vi "SwerveDrivePoseEst_AddVisionMeasurement.vi"(9 "TImeStamp_Seconds":dbl=0.02, 10 "visionRobotPose":T10={"TRANSLATION"={"X"=0.0, "Y"=0.0}, "ROTATION"={"VALUE"=0.0, "COS"=1.0, "SIN"=0.0}} {"ROTATION"."SIN" format="%13.4f"; "ROTATION"."COS" format="%13.4f"; "ROTATION"."VALUE" format="%13.4f"; "TRANSLATION"."Y" format="%14.3f"; "TRANSLATION"."X" format="%14.3f"}, 11 "in SwerveDrivePoseEstimate":T2={"M_VisionContR"=[], "m_nominal_dT"=0.0, "m_PrevTime_Sec"=0.0, "m_GyroOffset"={"VALUE"=0.0, "COS"=1.0, "SIN"=0.0}, "m_PrevAngle"={"VALUE"=0.0, "COS"=1.0, "SIN"=0.0}, "m_Observer"={"m_P"=[], "m_xHat"=[], "States"=0, "Outputs"=0, "m_ContR"=[], "m_ContQ"=[], "m_SigmasF"=[], "m_dT_Sec"=0.0, "MERWE_SCALED_SIGMA_PTS"={"m_Wm"=[], "States"=0, "Alpha"=0.0, "m_Wc"=[], "Kappa"=0}, "meanFuncX"=refnum, "meanFuncY"=refnum, "residualFuncX"=refnum, "residualFuncY"=refnum, "addFuncX"=refnum, "addFuncXExtra"=variant, "residualFuncYExtra"=variant, "residualFuncXExtra"=variant, "MeanFuncYExtra"=variant, "MeanFuncXExtra"=variant, "Inputs"=0}, "m_kinematics"={"NumModules"=0, "InverseKinematics"=[], "ForwardKinematics"=[], "Modules"=[], "PrevCoR"={"X"=0.0, "Y"=0.0}}, "Pose_Buffer"={"TimeStamps"=[], "Pose"=[], "Min_TimeStamp"=0.0, "Max_TimeStamp"=0.0, "ItemCount"=0, "MaxBufferTime"=0.0}} {"Pose_Buffer"."Pose"."ROTATION"."SIN" format="%13.4f"; "Pose_Buffer"."Pose"."ROTATION"."COS" format="%13.4f"; "Pose_Buffer"."Pose"."ROTATION"."VALUE" format="%13.4f"; "Pose_Buffer"."Pose"."TRANSLATION"."Y" format="%14.3f"; "Pose_Buffer"."Pose"."TRANSLATION"."X" format="%14.3f"; "m_kinematics"."PrevCoR"."Y" format="%14.3f"; "m_kinematics"."PrevCoR"."X" format="%14.3f"; "m_kinematics"."Modules"."Y" format="%14.3f"; "m_kinematics"."Modules"."X" format="%14.3f"; "m_PrevAngle"."SIN" format="%13.4f"; "m_PrevAngle"."COS" format="%13.4f"; "m_PrevAngle"."VALUE" format="%13.4f"; "m_GyroOffset"."SIN" format="%13.4f"; "m_GyroOffset"."COS" format="%13.4f"; "m_GyroOffset"."VALUE" format="%13.4f"}) -> (0 "Error":bool, 3 "OutSwerveDrivePoseEstimate":T2={"M_VisionContR"=[], "m_nominal_dT"=0.0, "m_PrevTime_Sec"=0.0, "m_GyroOffset"={"VALUE"=0.0, "COS"=1.0, "SIN"=0.0}, "m_PrevAngle"={"VALUE"=0.0, "COS"=1.0, "SIN"=0.0}, "m_Observer"={"m_P"=[], "m_xHat"=[], "States"=0, "Outputs"=0, "m_ContR"=[], "m_ContQ"=[], "m_SigmasF"=[], "m_dT_Sec"=0.0, "MERWE_SCALED_SIGMA_PTS"={"m_Wm"=[], "States"=0, "Alpha"=0.0, "m_Wc"=[], "Kappa"=0}, "meanFuncX"=refnum, "meanFuncY"=refnum, "residualFuncX"=refnum, "residualFuncY"=refnum, "addFuncX"=refnum, "addFuncXExtra"=variant, "residualFuncYExtra"=variant, "residualFuncXExtra"=variant, "MeanFuncYExtra"=variant, "MeanFuncXExtra"=variant, "Inputs"=0}, "m_kinematics"={"NumModules"=0, "InverseKinematics"=[], "ForwardKinematics"=[], "Modules"=[], "PrevCoR"={"X"=0.0, "Y"=0.0}}, "Pose_Buffer"={"TimeStamps"=[], "Pose"=[], "Min_TimeStamp"=0.0, "Max_TimeStamp"=0.0, "ItemCount"=0, "MaxBufferTime"=0.0}} {"Pose_Buffer"."Pose"."ROTATION"."SIN" format="%13.4f"; "Pose_Buffer"."Pose"."ROTATION"."COS" format="%13.4f"; "Pose_Buffer"."Pose"."ROTATION"."VALUE" format="%13.4f"; "Pose_Buffer"."Pose"."TRANSLATION"."Y" format="%14.3f"; "Pose_Buffer"."Pose"."TRANSLATION"."X" format="%14.3f"; "m_kinematics"."PrevCoR"."Y" format="%14.3f"; "m_kinematics"."PrevCoR"."X" format="%14.3f"; "m_kinematics"."Modules"."Y" format="%14.3f"; "m_kinematics"."Modules"."X" format="%14.3f"; "m_PrevAngle"."SIN" format="%13.4f"; "m_PrevAngle"."COS" format="%13.4f"; "m_PrevAngle"."VALUE" format="%13.4f"; "m_GyroOffset"."SIN" format="%13.4f"; "m_GyroOffset"."COS" format="%13.4f"; "m_GyroOffset"."VALUE" format="%13.4f"})   [LabVIEW 2019, in "Trajectory_Library.lvlib"]
doc: "Add a vision measurement to the Unscented Kalman Filter. This will correct the odometry pose estimate while still accounting for measurement noise.\n \nThis method can be called as infrequently as you want, as long as you are calling SwerveDrivePoseEstimator_update every loop.\n\nTo promote stability of the pose estimate and make it robust to bad vision data, we recommend only adding vision measurements that are already within one meter or so of the current pose estimate.\n \nInputs:\n - SwervePoseEst -- Data cluster containing SwervePoseEst data\n - visionRobotPoseMeters -- The pose of the robot as measured \n by the vision camera.\n - timestampSeconds -- The timestamp of the vision measurement in \n seconds. Note that if you don't use your own time \n source by calling SwerveDrivePoseEstimator_updateWithTime\n then you must use a timestamp with an epoch since FPGA \n startup (i.e. the epoch of this timestamp is the same \n epoch as Timer.getFPGATimestamp.) This means that you \n should use Timer.getFPGATimestamp as your time source or \n sync the epochs.\n\nOutputs:\n - outSwevePoseEst -- Updated data cluster \n - Error -- If TRUE, an error occured."
uses:
  Trajectory_Library.lvlib
  SWERVE_DRIVE_POSE_EST.ctl
  <vilib>/Analysis/Matrix/Datatypes/RealMatrix.ctl
  ROTATION2D.ctl
  UNSCENTED_KALMAN_FILTER.ctl
  MERWE_SCALED_SIGMA_PTS.ctl
  CALLBACK_FUNC_TYPE.ctl
  SWERVE_DRIVE_KINEMATICS.ctl
  TRANSLATION2D.ctl
  TIME_INTERPOLATABLE_POSE.ctl
  POSE2D.ctl
  Pose2d_RelativeTo.vi
  Transform2d_Create_TransRot.vi
  Translation2d_RotateBy.vi
  Translation2d_Plus.vi
  Rotation2d_Plus.vi
  Pose2d_New_TRRO.vi
  VecBuilder_3x1Fill.vi
  Pose2d_getXYAngle.vi
  Transform2d_Create_PosePose.vi
  Translation2d_Create.vi
  Rotation2d_RotateBy.vi
  Rotation2d_UnaryMinus.vi
  Translation2d_Minus.vi
  Rotation2d_Minus.vi
  Rotation2d_CreateXY.vi
  Rotation2d_CreateAngle.vi
  Util_CalcDist.vi
  <vilib>/Analysis/Matrix/NI_Matrix.lvlib
panel:
  in  "Cluster":cluster{"VisionDiscreteR":T1}
  # "<3, 3>"
  # "State Estimate <Statess,1>"
  # "<States, States>"
  # "<States, ?>"
  # "<Statess,  States>"
  # "<Outputs, Outputs>"
  # "<?, 1>"
  # "<?, 1>"
  # "<3, 3>"
  # "State Estimate <Statess,1>"
  # "<States, States>"
  # "<States, ?>"
  # "<Statess,  States>"
  # "<Outputs, Outputs>"
  # "<?, 1>"
  # "<?, 1>"
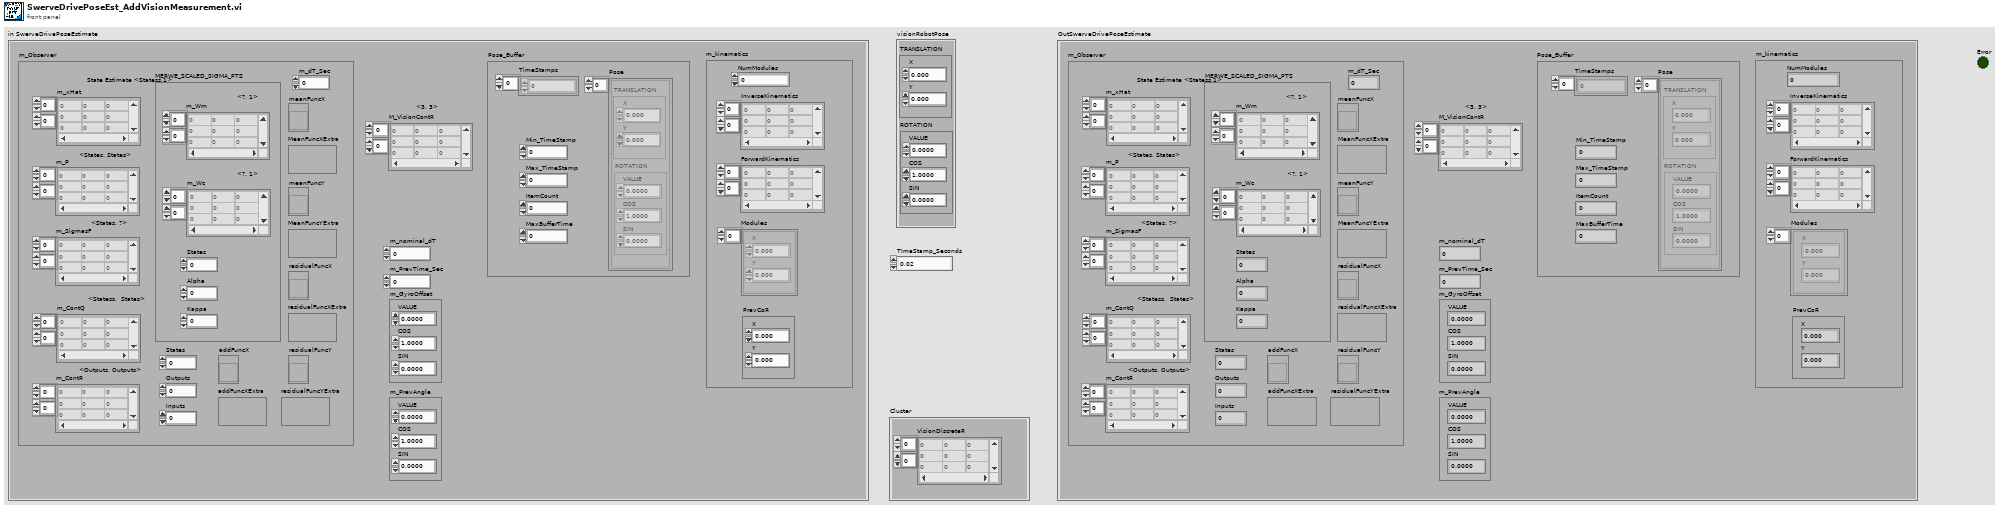
[diagram p1: front panel]
types:
  T1 = typedef "NI_Matrix.lvlib/RealMatrix.ctl" = dbl[][]
  T2 = typedef "Trajectory_Library.lvlib/SWERVE_DRIVE_POSE_EST.ctl" = cluster{"M_VisionContR":T1, "m_nominal_dT":dbl, "m_PrevTime_Sec":dbl, "m_GyroOffset":T3, "m_PrevAngle":T3, "m_Observer":T4, "m_kinematics":T7, "Pose_Buffer":T9}
  T3 = typedef "Trajectory_Library.lvlib/ROTATION2D.ctl" = cluster{"VALUE":dbl, "COS":dbl, "SIN":dbl}
  T4 = typedef "Trajectory_Library.lvlib/UNSCENTED_KALMAN_FILTER.ctl" = cluster{"m_P":T1, "m_xHat":T1, "States":i32, "Outputs":i32, "m_ContR":T1, "m_ContQ":T1, "m_SigmasF":T1, "m_dT_Sec":dbl, "MERWE_SCALED_SIGMA_PTS":T5, "meanFuncX":T6, "meanFuncY":T6, "residualFuncX":T6, "residualFuncY":T6, "addFuncX":T6, "addFuncXExtra":variant, "residualFuncYExtra":variant, "residualFuncXExtra":variant, "MeanFuncYExtra":variant, "MeanFuncXExtra":variant, "Inputs":i32}
  T5 = typedef "Trajectory_Library.lvlib/MERWE_SCALED_SIGMA_PTS.ctl" = cluster{"m_Wm":T1, "States":i32, "Alpha":dbl, "m_Wc":T1, "Kappa":i32}
  T6 = typedef "Trajectory_Library.lvlib/CALLBACK_FUNC_TYPE.ctl" = refnum<vi>
  T7 = typedef "Trajectory_Library.lvlib/SWERVE_DRIVE_KINEMATICS.ctl" = cluster{"NumModules":i32, "InverseKinematics":T1, "ForwardKinematics":T1, "Modules":T8[], "PrevCoR":T8}
  T8 = typedef "Trajectory_Library.lvlib/TRANSLATION2D.ctl" = cluster{"X":dbl, "Y":dbl}
  T9 = typedef "Trajectory_Library.lvlib/TIME_INTERPOLATABLE_POSE.ctl" = cluster{"TimeStamps":dbl[], "Pose":T10[], "Min_TimeStamp":dbl, "Max_TimeStamp":dbl, "ItemCount":i32, "MaxBufferTime":dbl}
  T10 = typedef "Trajectory_Library.lvlib/POSE2D.ctl" = cluster{"TRANSLATION":T8, "ROTATION":T3}
  T11 = typedef "Trajectory_Library.lvlib/TRANSFORM2D.ctl" = cluster{"TRANSLATION":T8, "ROTATION":T3}
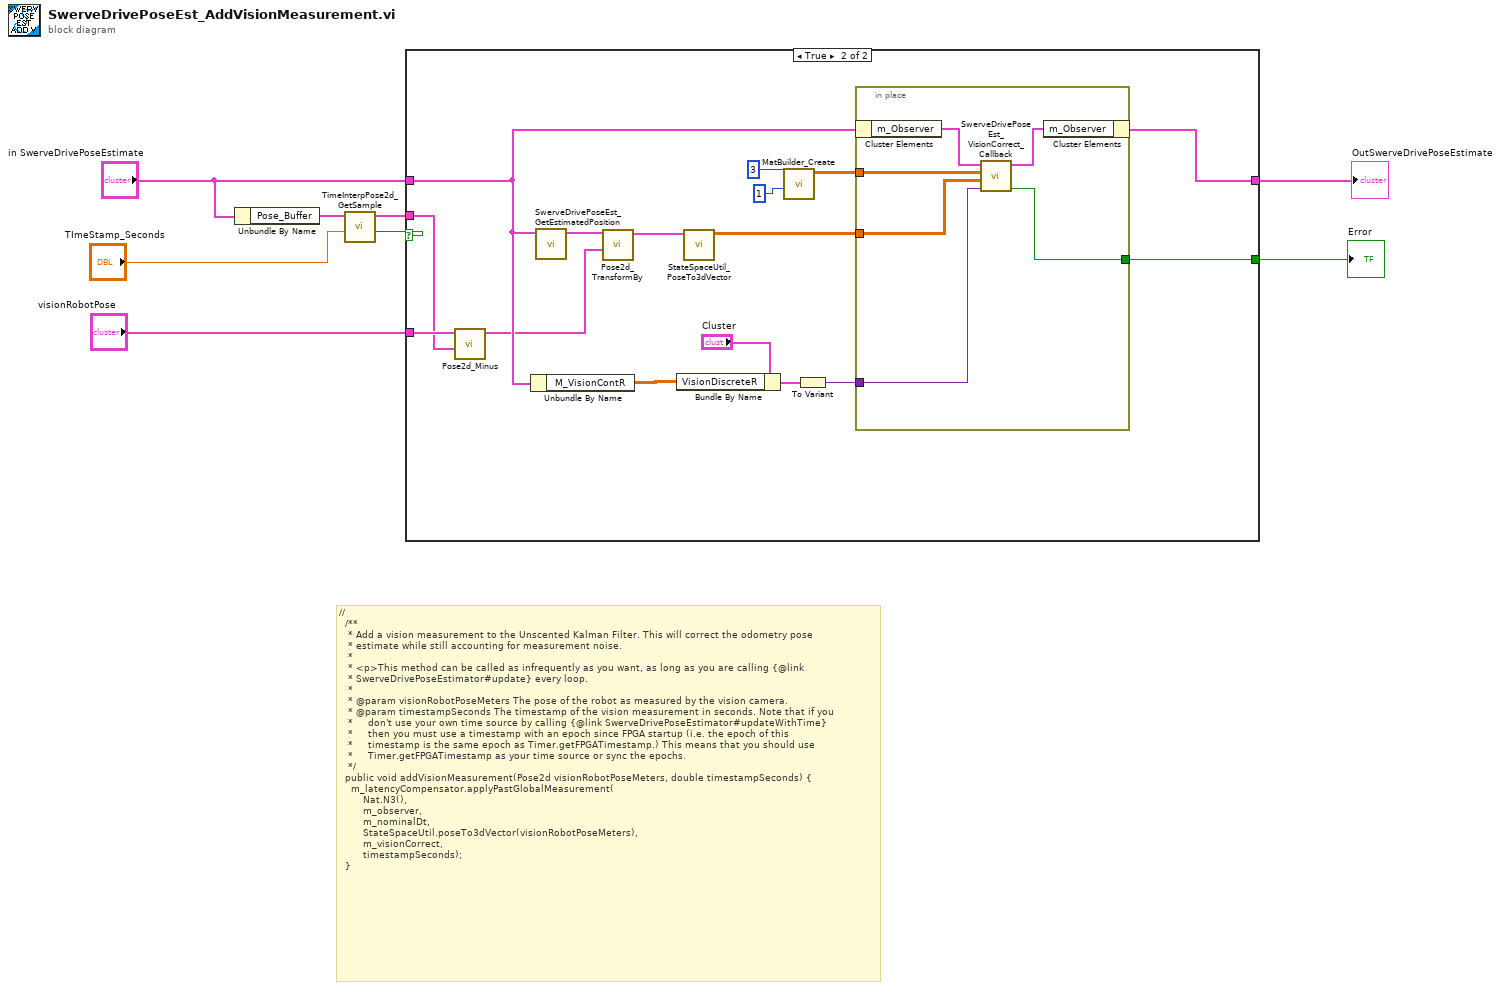
[diagram p0: block diagram]
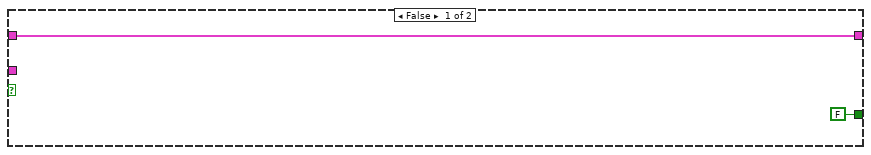
[diagram p2: hidden frame]
diagram:
  # "// \n  /**\n   * Add a vision measurement to the Unscented Kalman Filter. This will correct the odometry pose\n   * estimate while still accounting for measurement noise.\n   *\n   * <p>This method can be called as infrequently as you want, as long as you are calling {@link\n   * SwerveDrivePoseEstimator#update} every loop.\n   *\n   * @param visionRobotPoseMeters The pose of the robot as measured by the vision camera.\n   * @param timestampSeconds The timestamp of the vision measurement in seconds. Note that if you\n   *     don't use your own time source by calling {@link SwerveDrivePoseEstimator#updateWithTime}\n   *     then you must use a timestamp with an epoch since FPGA startup (i.e. the epoch of this\n   *     timestamp is the same epoch as Timer.getFPGATimestamp.) This means that you should use\n   *     Timer.getFPGATimestamp as your time source or sync the epochs.\n   */\n  public void addVisionMeasurement(Pose2d visionRobotPoseMeters, double timestampSeconds) {\n    m_latencyCompensator.applyPastGlobalMeasurement(\n        Nat.N3(),\n        m_observer,\n        m_nominalDt,\n        StateSpaceUtil.poseTo3dVector(visionRobotPoseMeters),\n        m_visionCorrect,\n        timestampSeconds);\n  }"
  n1 = Unbundle By Name("in SwerveDrivePoseEstimate") -> ("Pose_Buffer"=w8:T9)
  n2 = call "TimeInterpPose2d_GetSample.vi"("TimeStamp"="TImeStamp_Seconds", "TimeInterpPose"=w8) -> ("IsPresent"=w6:bool, "OutputPose"=w7:T10)  [unwired: 8 in]
  n3 = case shown="True" w6 {
    tunnel: [w10 w26] -> w2
    tunnel: "visionRobotPose" -> [_ w23]
    tunnel: [FALSE w20] -> w1
    tunnel: "in SwerveDrivePoseEstimate" -> [w10 w25]
    tunnel: w7 -> [_ w22]
    frame False {
    }
    frame True {
      n4 = call "Pose2d_Minus.vi"("other TRANSFORM"=w22, "in POSE"=w23) -> ("outTRANSFORM"=w21:T11)  [unwired: 9 in]
      n5 = Unbundle By Name(w25) -> ("M_VisionContR"=w14:T1)
      n6 = call "SwerveDrivePoseEst_GetEstimatedPosition.vi"("in SwerveDrivePoseEstimate"=w25) -> ("Estimated Pose"=w24:T10)  [unwired: 10 in]
      n7 = call "Pose2d_TransformBy.vi"("other TRANSFORM"=w21, "in POSE"=w24) -> ("out POSE"=w12:T10)  [unwired: 9 in]
      n8 = Bundle By Name(cluster="Cluster", "VisionDiscreteR"=w14) -> (w15:cluster{"VisionDiscreteR":T1})
      n9 = call "StateSpaceUtil_PoseTo3dVector.vi"("Pose"=w12) -> ("Pose Vector"=w11:T1)  [unwired: 10 in]
      n10 = call "MatBuilder_Create.vi"("Columns"=1, "Rows"=3) -> ("output matrix"=w17:T1)  [unwired: 9 in]
      n11 = To Variant(anything=w15) -> (Variant=w13:variant)
      n12 = in-place {
        in-place-border: [w30] -> w20
        in-place-border: w17 -> [w29]
        in-place-border: w13 -> [w28]
        in-place-border: w11 -> [w27]
        n13 = in-place-cluster #1(w25) -> ("m_Observer"=w32:T4)
        n14 = call "SwerveDrivePoseEst_VisionCorrect_Callback.vi"("ExtraPassedData"=w28, "Y"=w27, "U"=w29, "in UNSCENTED_KALMAN_FILTER"=w32) -> ("Error"=w30:bool, "out UNSCENTED_KALMAN_FILTER"=w31:T4)  [unwired: 6 in]
        n15 = in-place-cluster #1("m_Observer"=w31) -> (w26:T2)
      }
    }
  }
  "OutSwerveDrivePoseEstimate" <- w2
  "Error" <- w1
